vi "limit speed (SubVI).vi"(7 "enable":bool=TRUE, 11 "keypad cmd":string) -> (3 "keypad cmd  out":string)   [LabVIEW 2018]
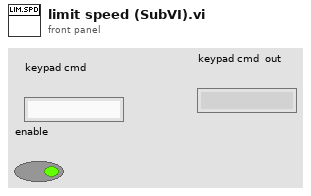
[diagram p1: front panel]
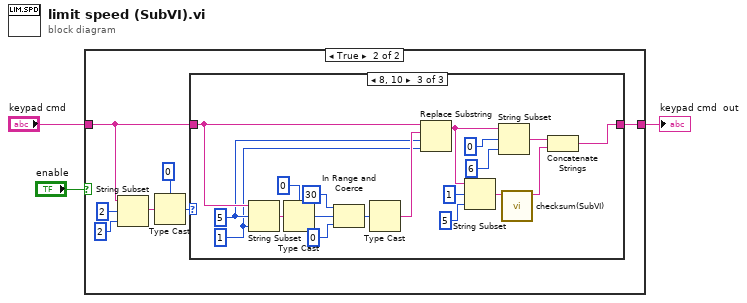
[diagram p0: block diagram]
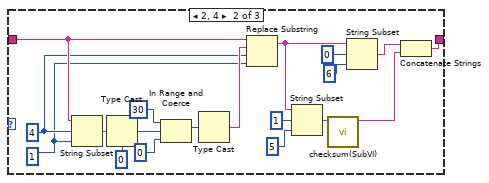
[diagram p4: hidden frame]
diagram:
  n1 = case shown="True" "enable" {
    tunnel: "keypad cmd" -> [w4 w6]
    tunnel: [w4 w5] -> w2
    frame False {
    }
    frame True {
      n2 = String Subset(string=w6, offset (0)=2, length (rest)=2 ("length (rest)")) -> (substring=w9:string)
      n3 = Type Cast(type=u16 0, x=w9) -> (*(type *) &x=w7:u16)
      n4 = case shown="8, 10" w7 {
        tunnel: w6 -> [w12 w26 w45]
        tunnel: [w12 w13 w32] -> w5
        frame 0, Default {
        }
        frame 2, 4 {
          w22 = 1 ("length (rest)")
          w23 = 4 ("offset (0)")
          n5 = String Subset(string=w26, offset (0)=w23, length (rest)=w22) -> (substring=w31:string)
          n6 = Type Cast(type=u8 0, x=w31) -> (*(type *) &x=w29:u8)
          n7 = In Range and Coerce(upper limit=u8 30, x=w29, lower limit=u8 0) -> (coerced(x)=w25:u8)  [unwired: 1 out]
          n8 = Type Cast(x=w25) -> (*(type *) &x=w24:string)  [unwired: 1 in]
          n9 = Replace Substring(2:w22, 3:w23, 4:w24, 5:w26) -> (1:w14:string)  [unwired: 1 out]
          n10 = String Subset(string=w14, offset (0)=1, length (rest)=5 ("length (rest)")) -> (substring=w19:string)
          n11 = call "checksum(SubVI).vi"("response"=w19) -> ("CHKSUM"=w16:string)  [unwired: 10 in]
          n12 = String Subset(string=w14, offset (0)=0, length (rest)=6 ("length (rest)")) -> (substring=w15:string)
          n13 = Concatenate Strings(w15, w16) -> (w13:string)
        }
        frame 8, 10 {
          w41 = 1 ("length (rest)")
          w42 = 5 ("offset (0)")
          n14 = String Subset(string=w45, offset (0)=w42, length (rest)=w41) -> (substring=w50:string)
          n15 = Type Cast(type=u8 0, x=w50) -> (*(type *) &x=w48:u8)
          n16 = In Range and Coerce(upper limit=u8 30, x=w48, lower limit=u8 0) -> (coerced(x)=w44:u8)  [unwired: 1 out]
          n17 = Type Cast(x=w44) -> (*(type *) &x=w43:string)  [unwired: 1 in]
          n18 = Replace Substring(2:w41, 3:w42, 4:w43, 5:w45) -> (1:w35:string)  [unwired: 1 out]
          n19 = String Subset(string=w35, offset (0)=1, length (rest)=5 ("length (rest)")) -> (substring=w38:string)
          n20 = String Subset(string=w35, offset (0)=0, length (rest)=6 ("length (rest)")) -> (substring=w33:string)
          n21 = call "checksum(SubVI).vi"("response"=w38) -> ("CHKSUM"=w34:string)  [unwired: 10 in]
          n22 = Concatenate Strings(w33, w34) -> (w32:string)
        }
      }
    }
  }
  "keypad cmd  out" <- w2
